vi "AutoDecoder.vi"(10 "index":i32, 11 "Input Array":string[](array[string])) -> (2 "Tenths of Sec":i32, 3 "Case":string)   [LabVIEW 2016]
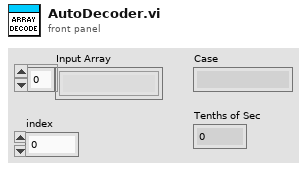
[diagram p1: front panel]
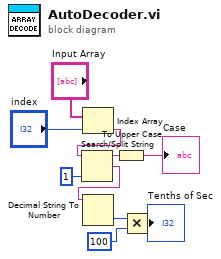
[diagram p0: block diagram]
diagram:
  n1 = Index Array(array="Input Array", index="index") -> (element=w4:string)
  n2 = Search/Split String(string=w4, offset (0)=1) -> (substring before match=w10:string, match + rest of string=w6:string)  [unwired: 1 in, 1 out]
  n3 = Decimal String To Number(string=w6) -> (number=w7:i32)  [unwired: 2 in, 1 out]
  n4 = To Upper Case(1:w10) -> (0:→"Case":string)
  n5 = Multiply(x=w7, y=100) -> (x*y=→"Tenths of Sec":i32)
